vi "FlatToRichni_xnet_can_bm_api_PassThruRequest.vi"(5 "OutputClusterType":T1, 11 "InputCluster":T3) -> (3 "OutputCluster":T1)   [LabVIEW 2025, in "xnet_can_bus_monitor_api_server.lvlib"]
uses:
  xnet_can_bus_monitor_api_server.lvlib
  ni_xnet_can_bm_api_PassThruRequest_Flat.ctl
  ni_xnet_can_bm_api_Frame_Flat.ctl
  ni_xnet_can_bm_api_PassThruRequest.ctl
  ni_xnet_can_bm_api_Frame.ctl
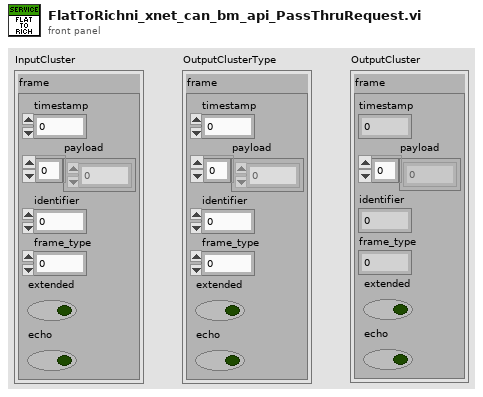
[diagram p1: front panel]
types:
  T1 = typedef "xnet_can_bus_monitor_api_server.lvlib/ni_xnet_can_bm_api_PassThruRequest.ctl" = cluster{"frame":T2}
  T2 = typedef "xnet_can_bus_monitor_api_server.lvlib/ni_xnet_can_bm_api_Frame.ctl" = cluster{"timestamp":dbl, "payload":u8[], "identifier":u32, "frame_type":u32, "extended":bool, "echo":bool}
  T3 = typedef "xnet_can_bus_monitor_api_server.lvlib/ni_xnet_can_bm_api_PassThruRequest_Flat.ctl" = cluster{"frame":T4}
  T4 = typedef "xnet_can_bus_monitor_api_server.lvlib/ni_xnet_can_bm_api_Frame_Flat.ctl" = cluster{"timestamp":dbl, "payload":u8[], "identifier":u32, "frame_type":u32, "extended":bool, "echo":bool}
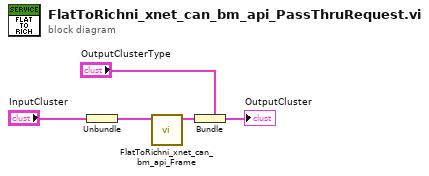
[diagram p0: block diagram]
diagram:
  n1 = Unbundle "Unbundle"("InputCluster") -> ("frame"=w2:T4)
  n2 = call "FlatToRichni_xnet_can_bm_api_Frame.vi"("InputCluster"=w2) -> ("OutputCluster"=w1:T2)  [unwired: 10 in]
  n3 = Bundle "Bundle"(cluster="OutputClusterType", "frame"=w1) -> (→"OutputCluster":T1)
